vi "USB4065 single measure.vi"(8 "error in (no error)":errorcluster, 9 "Configuration:Range":dbl=10.0, 10 "Configuration:Function":i32(ring)=1 items=["DC Volts"=1, "AC Volts"=2, "DC Current"=3, "AC Current"=4, "2-Wire Resistance"=5, "4-Wire Resistance"=101, "Frequency"=104, "Period"=105, "AC Volts DC Coupled"=1001, "Diode"=1002, "Waveform Voltage"=1003, "Waveform Current"=1004, "Capacitance"=1005, "Inductance"=1006, "Temperature"=108], 11 "Instrument Descriptor":refnum<k15>="Dev2") -> (0 "error out":errorcluster, 2 "Measurement":dbl format="%.12f", 3 "instrument handle out":refnum<k15>)   [LabVIEW 2009]
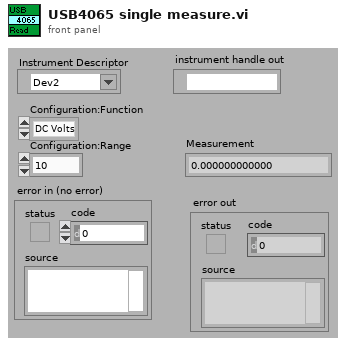
[diagram p1: front panel]
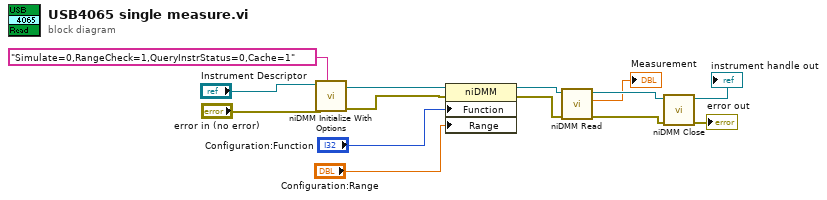
[diagram p0: block diagram]
diagram:
  n1 = call <instrlib>:"niDMM Initialize With Options.vi"("Option String"="Simulate=0,RangeCheck=1,QueryInstrStatus=0,Cache=1", "error in (no error)"="error in (no error)", "Instrument Descriptor"="Instrument Descriptor") -> ("error out"=w5:errorcluster, "instrument handle out"=w8:refnum<k15>)  [unwired: 2 in, 5 out]
  n2 = property class="niDMM"(reference=w8, error in=w5, "Function"="Configuration:Function", "Range"="Configuration:Range") -> (reference out=w6:refnum<k15>, error out=w4:errorcluster)
  n3 = call <instrlib>:"niDMM Read.vi"("error in (no error)"=w4, "instrument handle"=w6) -> ("error out"=w9:errorcluster, "Measurement"=→"Measurement":dbl, "instrument handle out"=w11:refnum<k15>)  [unwired: 1 in, 6 out]
  "instrument handle out" <- w11
  n4 = call <instrlib>:"niDMM Close.vi"("error in (no error)"=w9, "instrument handle"=w11) -> ("error out"=→"error out":errorcluster)  [unwired: 9 out]
